vi "Table, Find Row in Column.vi"(8 "error in":errorcluster, 9 "search key":string, 10 "search column (0)":i32, 11 "Tbl Refnum":refnum<vi>) -> (0 "error out":errorcluster, 1 "found":bool, 2 "row index":i32=-1, 3 "Tbl Refnum out":refnum<vi>)   [LabVIEW 2020]
doc: "Search a single column in a table to find a match and output the row index.\nIf the row index is less than zero, then no match was found."
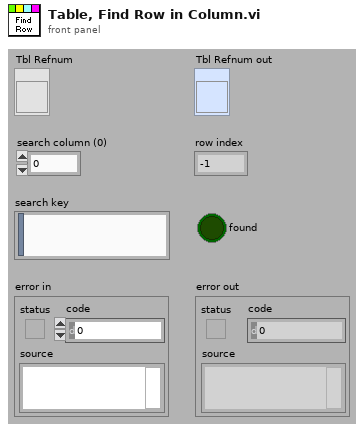
[diagram p1: front panel]
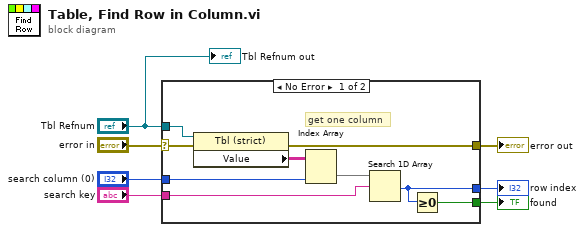
[diagram p0: block diagram]
diagram:
  n1 = case shown="No Error" "error in" {
    selector: "error in" -> [w14 w17]
    tunnel: "Tbl Refnum" -> [w16 _]
    tunnel: [w15 w17] -> w7
    tunnel: "search column (0)" -> [w8 _]
    tunnel: [w13 _] -> w3
    tunnel: [w12 _] -> w2
    tunnel: "search key" -> [w11 _]
    frame No Error {
      # "get one column"
      n2 = property class="Tbl (strict)"(reference=w16, error in=w14) -> (error out=w15:errorcluster, "Value"=w10:string[][])  [unwired: 1 out]
      n3 = Index Array(array=w10, index (col)=w8) -> (element=w9:string[])  [unwired: 1 in]
      n4 = Search 1D Array(1D array=w9, element=w11) -> (index of element=w13:i32)  [unwired: 1 in]
      n5 = Greater Or Equal To 0?(x=w13) -> (x >= 0?=w12:bool)
    }
    frame Error {
    }
  }
  "row index" <- w3
  "error out" <- w7
  "found" <- w2
  "Tbl Refnum out" <- "Tbl Refnum"
